vi "Lambda (SubVI).vi"() -> (3 "Lambda":dbl[](array[numeric]))   [LabVIEW 2019]
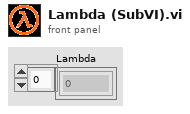
[diagram p1: front panel]
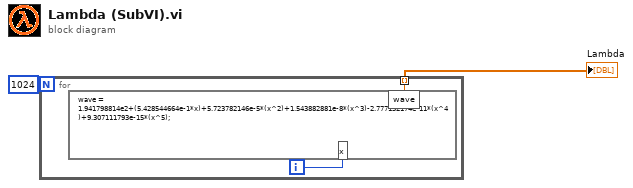
[diagram p0: block diagram]
diagram:
  n1 = for {
    N: 1024 -> [_]
    tunnel: [w3] -> w2 mode=indexing
    i -> [w4]
    n2 = formula code="wave = 1.941798814e2+(5.428544664e-1*x)+5.723782146e-5*(x^2)+1.543882881e-8*(x^3)-2.777152174e-11*(x^4)+9.307111793e-15*(x^5);"("x"=w4) -> ("wave"=w3:dbl)
  }
  "Lambda" <- w2
